vi "DDAQ-Get-Many.vi"(8 "error in (no error)":errorcluster, 9 "max bytes to read (10000)":i32=10000, 10 "SCPI-like Keywords (leave off question marks)":string[](array[string]), 11 "connection ID":refnum<k5>) -> (0 "error out":errorcluster, 1 "Query":string, 2 "Responses":string[](array[string]), 3 "connection ID out":refnum<k5>, 4 "Elapsed time, ms (debug)":u32)   [LabVIEW 2020]
panel:
  out "bytes written":i32
  out "Response":string
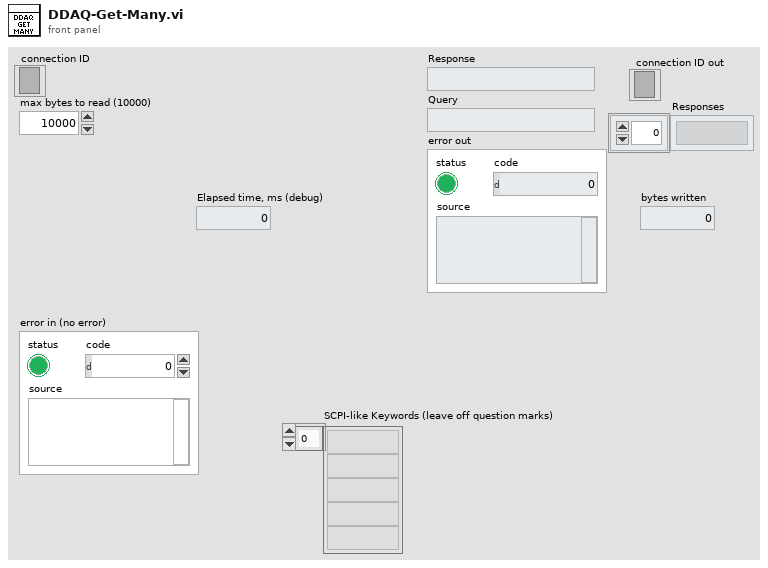
[diagram p1: front panel]
types:
  T1 = enum16{"Standard", "Buffered", "CRLF", "Immediate"}
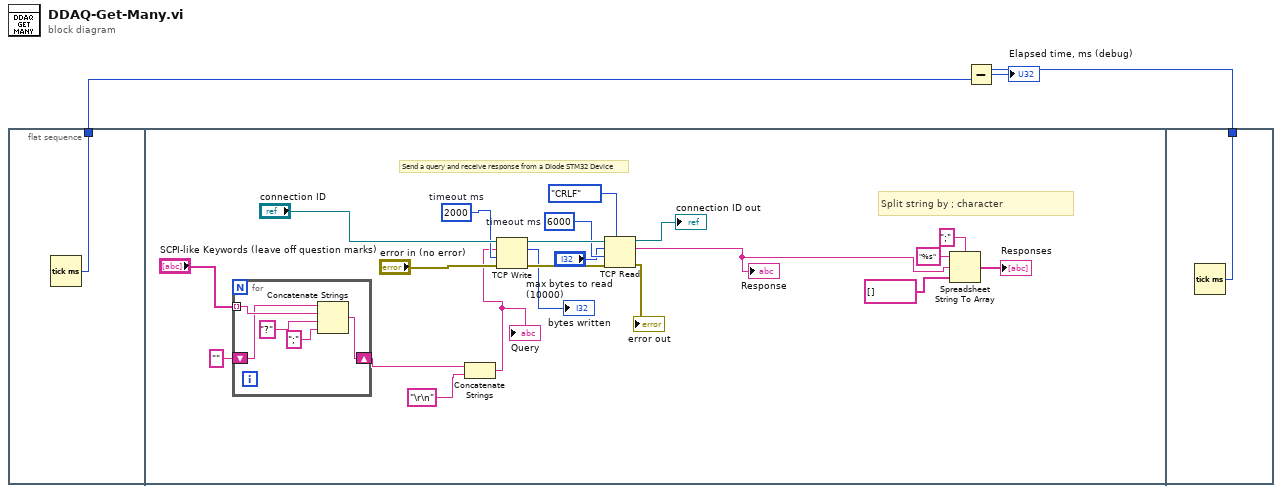
[diagram p0: block diagram]
diagram:
  n1 = flat-sequence {
    tunnel: [w4] -> w2
    tunnel: [w31] -> w3
    frame #0 {
      n2 = Tick Count (ms)() -> (millisecond timer value=w4:u32)
    }
    frame #1 {
      w16 = 6000  # timeout ms
      w17 = 2000  # timeout ms
      # "Split string by ; character"
      # "Send a query and receive response from a Diode STM32 Device"
      n3 = for {
        tunnel: "SCPI-like Keywords (leave off question marks)" -> [w29] mode=indexing
        shift-right: [w28] -> w12
        shift-left: "" -> [w26]
        n4 = Concatenate Strings(w26, w29, "?", ";" ("string")) -> (w28:string)
      }
      n5 = Concatenate Strings(w12, "\r\n") -> (w11:string)
      "Query" <- w11
      n6 = TCP Write(connection ID="connection ID", data in=w11, error in (no error)="error in (no error)", 9:w17) -> (connection ID out=w23:refnum<k5>, bytes written=→"bytes written":i32, error out=w22:errorcluster)
      n7 = TCP Read(connection ID=w23, bytes to read="max bytes to read (10000)", error in (no error)=w22, 7:T1."CRLF" ("mode (standard)"), 9:w16) -> (connection ID out=→"connection ID out":refnum<k5>, data out=w6:string, error out=→"error out":errorcluster)
      "Response" <- w6
      n8 = Spreadsheet String To Array(delimiter (Tab)=";", format string="%s", spreadsheet string=w6, array type (2D Dbl)=string[] []) -> (array=→"Responses":string[])
    }
    frame #2 {
      n9 = Tick Count (ms)() -> (millisecond timer value=w31:u32)
    }
  }
  n10 = Subtract(x=w3, y=w2) -> (x-y=→"Elapsed time, ms (debug)":u32)
